vi "update_attrs.vi"(8 "error in (no error)":errorcluster, 10 "Nested Enqueuers Map":T1(c390), 11 "Udate Nested Attributes in":refnum<class "Udate Nested Attributes.lvclass">) -> (0 "error out":errorcluster, 3 "Udate Nested Attributes out":refnum<class "Udate Nested Attributes.lvclass">)   [LabVIEW 2025, in "Udate Nested Attributes.lvclass"]
uses:
  Udate Nested Attributes.lvclass
  <vilib>/ActorFramework/Message Enqueuer/Message Enqueuer.lvclass
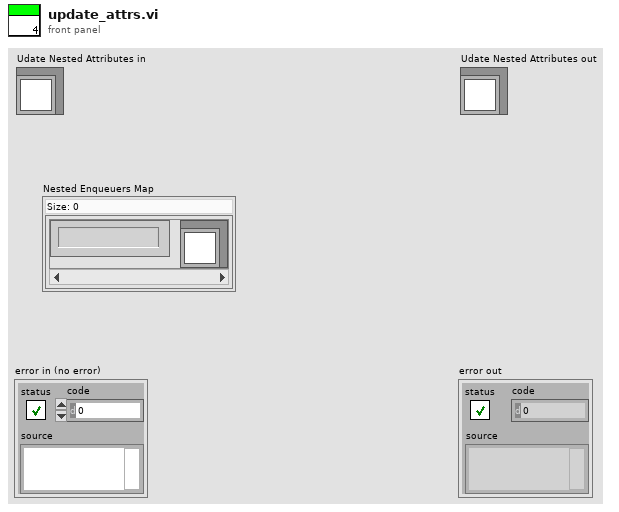
[diagram p1: front panel]
types:
  T1 = map{string, refnum<class "Message Enqueuer.lvclass">}
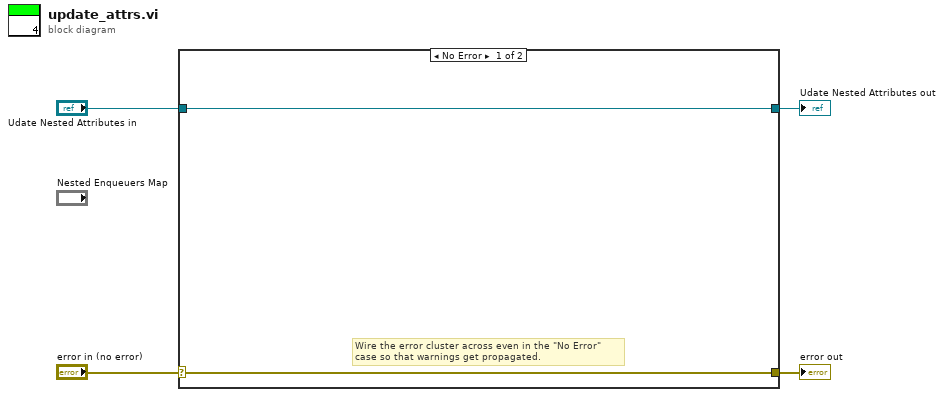
[diagram p0: block diagram]
diagram:
  n1 = case shown="No Error" "error in (no error)" {
    selector: "error in (no error)" -> [w5 w8]
    tunnel: [w5 w8] -> w3
    tunnel: [w6 w7] -> w1
    tunnel: "Udate Nested Attributes in" -> [w6 w7]
    frame No Error {
      # "Wire the error cluster across even in the \"No Error\"\ncase so that warnings get propagated."
    }
    frame Error {
    }
  }
  "error out" <- w3
  "Udate Nested Attributes out" <- w1
